vi "FGV_PSP - IPS120 Mode Status.vi"(4 "error in":errorcluster, 6 "Function":enum16{"write", "read"}(ring), 7 "Mode":T1) -> (0 "error out":errorcluster, 3 "Mode":T1)   [LabVIEW 2016, in "IPS-120.lvlib" / "IPS-120-API.lvlib"]
uses:
  IPS-120-API.lvlib
  IPS120/Typedefs/Read Mode 2 - Enum.ctl
  IPS-120.lvlib
panel:
  # "Disabled calls to PSP 4/13/2018"
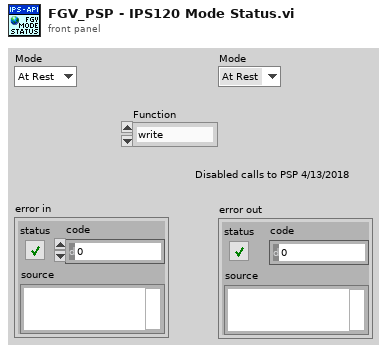
[diagram p1: front panel]
types:
  T1 = typedef "IPS-120.lvlib/Read Mode 2 - Enum.ctl" = enum16{"At Rest", "Sweeping", "Sweep Limiting", "Sweeping & Sweep Limiting"}
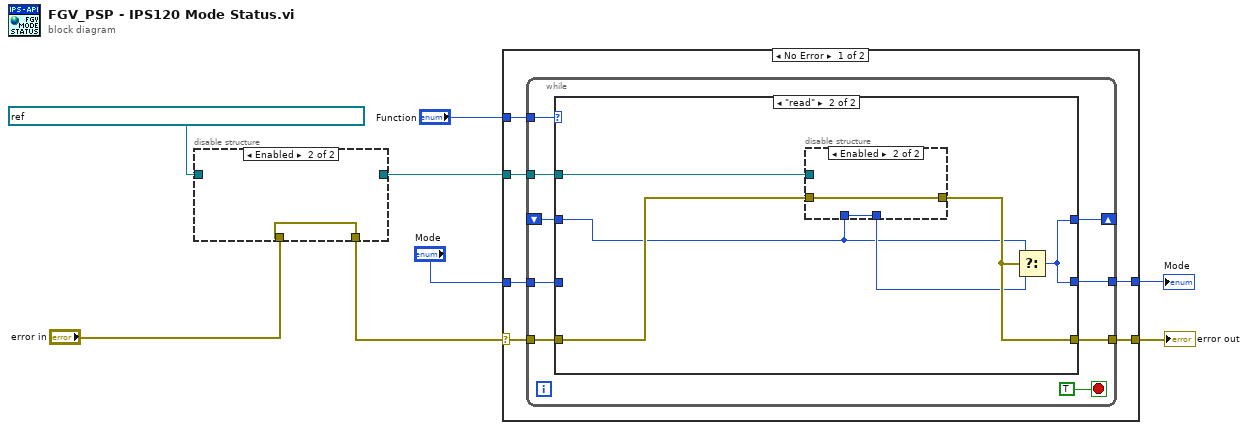
[diagram p0: block diagram]
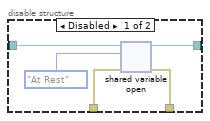
[diagram p2: hidden frame]
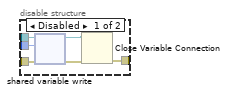
[diagram p4: hidden frame]
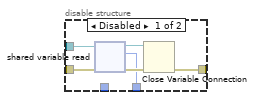
[diagram p5: hidden frame]
diagram:
  n1 = disable-structure shown="Enabled" {
    disable-tunnel: [w13 _] -> w6
    disable-tunnel: refnum<k21> "ni.var.psp://localhost/IPS120/ModeStatus" ("shared variable refnum in") -> [w12 _]
    disable-tunnel: [w11 w14] -> w4
    disable-tunnel: "error in" -> [w10 w14]
    frame Disabled {
      n2 = shared-variable-open(w12, w10, Read_Mode_2_-_Enum."At Rest" ("Mode 2")) -> (w13:refnum<k21>, w11:errorcluster)  [unwired: 1 in]
    }
    frame Enabled {
    }
  }
  n3 = case shown="No Error" w4 {
    selector: w4 -> [w20 w56]
    tunnel: [w19 w56] -> w8
    tunnel: [w18 w55] -> w1
    tunnel: "Function" -> [w17 _]
    tunnel: w6 -> [w16 _]
    tunnel: "Mode" -> [w15 w55]
    frame No Error {
      n4 = while {
        shift-right: [w24] -> _
        shift-left: _ -> [w23]
        tunnel: w20 -> [w28]
        tunnel: [w27] -> w19
        tunnel: [w26] -> w18
        tunnel: w17 -> [w25]
        tunnel: w16 -> [w22]
        tunnel: w15 -> [w21]
        stop <- TRUE stop-if-true
        n5 = case shown="\"read\"" w25 {
          tunnel: w28 -> [w32 w43]
          tunnel: [w33 w45] -> w27
          tunnel: [w30 w46] -> w26
          tunnel: [w30 w46] -> w24
          tunnel: w23 -> [_ w41]
          tunnel: w22 -> [w31 w44]
          tunnel: w21 -> [w30 _]
          frame "write", Default {
            n6 = disable-structure shown="Enabled" {
              disable-tunnel: [w38 w40] -> w33
              disable-tunnel: w32 -> [w36 w40]
              disable-tunnel: w31 -> [w35 _]
              disable-tunnel: w30 -> [w34 _]
              frame Disabled {
                n7 = shared-variable-write(w35, w36, w34) -> (w37:refnum<k21>, w39:errorcluster)
                n8 = Close Variable Connection(8:w39, 11:w37) -> (0:w38:errorcluster)
              }
              frame Enabled {
              }
            }
          }
          frame "read" {
            n9 = disable-structure shown="Enabled" {
              disable-tunnel: [w50 w53] -> w45
              disable-tunnel: w44 -> [w49 _]
              disable-tunnel: w43 -> [w48 w53]
              disable-tunnel: [w47 w54] -> w42
              disable-tunnel: w41 -> [_ w54]
              frame Disabled {
                n10 = shared-variable-read(w49, w48) -> (w52:refnum<k21>, w51:errorcluster, w47:T1)  [unwired: 1 out]
                n11 = Close Variable Connection(8:w51, 11:w52) -> (0:w50:errorcluster)
              }
              frame Enabled {
              }
            }
            n12 = Select(t=w41, s=w45, f=w42) -> (s? t:f=w46:T1)
          }
        }
      }
    }
    frame Error {
    }
  }
  "error out" <- w8
  "Mode" <- w1
